vi "Stop Configure UI.vi"(8 "error in (no error)":errorcluster, 9 "Configure VI Refnum":refnum<vi>, 10 "Container":refnum<vi>, 11 "SerializableObject in":refnum<class "SerializableObject.lvclass">) -> (0 "error out":errorcluster, 3 "SerializableObject out":refnum<class "SerializableObject.lvclass">)   [LabVIEW 2015, in "Editor.lvclass"]
uses:
  Editor.lvclass
  SerializableObject/SerializableObject.lvclass
  Project.lvclass
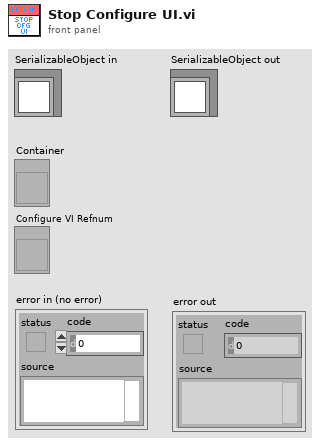
[diagram p1: front panel]
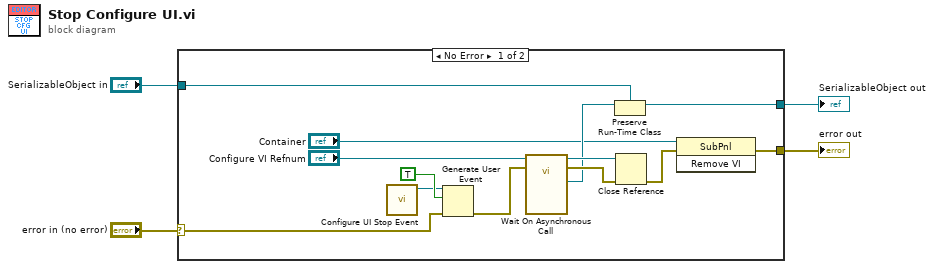
[diagram p0: block diagram]
diagram:
  n1 = case shown="No Error" "error in (no error)" {
    selector: "error in (no error)" -> [w16 w19]
    tunnel: [w12 w19] -> w3
    tunnel: [w9 w18] -> w1
    tunnel: "SerializableObject in" -> [w11 w18]
    frame No Error {
      n2 = call "Configure UI Stop Event.vi"() -> ("UI Stop event"=w7:refnum<user-event>)  [unwired: 11 in]
      n3 = Generate User Event(user event=w7, event data cluster=TRUE, error in=w16) -> (error out=w15:errorcluster)  [unwired: 1 in, 1 out]
      n4 = call-by-ref "Wait On Asynchronous Call"(reference="Configure VI Refnum", error in=w15) -> (reference out=w14:refnum<vi>, error out=w13:errorcluster, "SerializableObject out"=w10:refnum<class>)  [unwired: 10 in, 1 out]
      n5 = Preserve Run-Time Class(object in=w10, 2:w11) -> (object out=w9:refnum<class "SerializableObject.lvclass">)  [unwired: 1 in, 1 out]
      n6 = Close Reference(reference=w14, error in (no error)=w13) -> (error out=w8:errorcluster)
      n7 = invoke class="SubPnl" method="Remove VI"(reference="Container", error in=w8) -> (error out=w12:errorcluster)  [unwired: 1 in, 2 out]
    }
    frame Error {
    }
  }
  "error out" <- w3
  "SerializableObject out" <- w1
